vi "GEOM_GetROI.vi"(8 "error in (no error)":errorcluster) -> (0 "error out":errorcluster, 2 "Requested ROI":string)   [LabVIEW 2016]
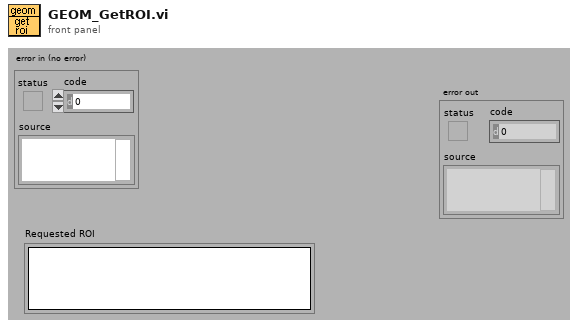
[diagram p1: front panel]
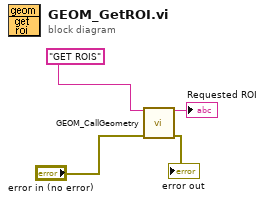
[diagram p0: block diagram]
diagram:
  n1 = call "GEOM_CallGeometry.vi"("Command"="GET ROIS", "error in (no error)"="error in (no error)") -> ("ImmedReplyString"=→"Requested ROI":string, "error out"=→"error out":errorcluster)  [unwired: 12 out]
